vi "Build VCOM Signal Lookup.vi"(8 "Error in":errorcluster, 11 "VCOM config file in":path=path "C:/Users/Public/Documents/National Instruments/NI-VCOM/configuration/Single_Point/CAN/VCOMConfig.xml") -> (0 "Error out":errorcluster, 2 "VCOM signal list":T1[](array[typedef]), 3 "VCOM Signal Map":map{string, T1}(c390))   [LabVIEW 2025]
uses:
  <vilib>/Vehicle Communication Toolkit/TypDefs/RBS Signal.ctl
  <vilib>/Vehicle Communication Toolkit/Full.lvlib
  <vilib>/Vehicle Communication Toolkit/Vehicle Communication Toolkit.lvlib
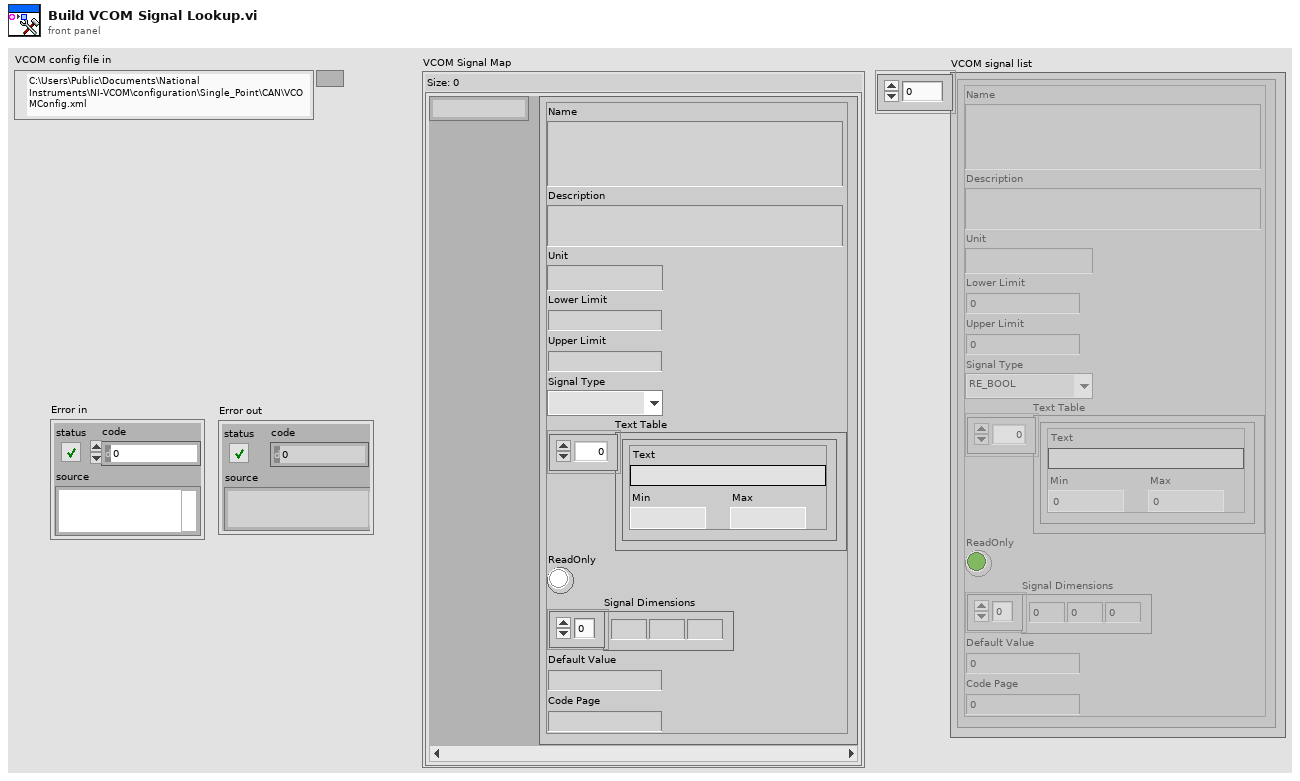
[diagram p1: front panel]
types:
  T1 = typedef "Vehicle Communication Toolkit.lvlib/RBS Signal.ctl" = cluster{"Name":string, "Description":string, "Unit":string, "Lower Limit":dbl, "Upper Limit":dbl, "Signal Type":enum32{"RE_BOOL", "RE_UINT8", "RE_INT8", "RE_UINT16", "RE_INT16", "RE_UINT32", "RE_INT32", "RE_UINT64", "RE_INT64", "RE_FLOAT32", "RE_FLOAT64", "RE_TEXT"}, "Text Table":cluster{"Text":string, "Min":dbl, "Max":dbl}[], "ReadOnly":bool, "Signal Dimensions":u32[], "Default Value":dbl, "Code Page":u32}
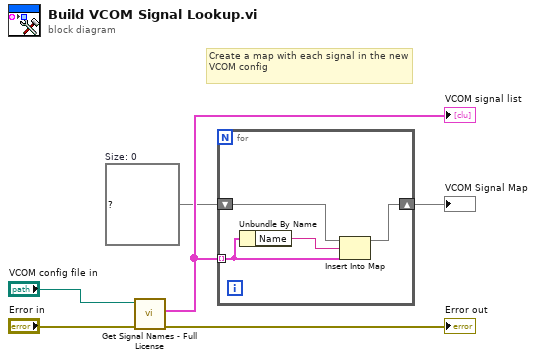
[diagram p0: block diagram]
diagram:
  w4 = map{string, T1} {}  # Size: 0
  # "Create a map with each signal in the new VCOM config"
  n1 = call <vilib>:"Get Signal Names - Full License.vi"("Error in"="Error in", "VCOM config file in"="VCOM config file in") -> ("Error out"=→"Error out":errorcluster, "VCOM signal list"=w5:T1[])  [unwired: 7 in, 1 out]
  "VCOM signal list" <- w5
  n2 = for {
    tunnel: w5 -> [w10] mode=indexing
    shift-right: [w7] -> w2
    shift-left: w4 -> [w8]
    n3 = Unbundle By Name(w10) -> ("Name"=w9:string)
    n4 = Insert Into Map(map in=w8, key=w9, value=w10) -> (map out=w7:map{string, T1})  [unwired: 2 out]
  }
  "VCOM Signal Map" <- w2
